vi "Create Case Structure.vi"(6 "Mouse Position":T1, 7 "User VI Ref":refnum<vi>, 8 "Is Multi-select?":bool, 9 "Remaining Items":refnum<vi>[](array[refnum]), 10 "Affected Items":T8, 11 "Menu Refnum":refnum<k9>) -> (3 "Menu Items To Add":T2[](array[typedef]))   [LabVIEW 2024]
doc: "This VI is part of a plug-in for modifying the LabVIEW shortcut menus. This is the builder VI which is called when the shortcut menu is built. It tells LabVIEW which shortcut menu items to add to the menu."
uses:
  <resource>/plugins/PopupMenus/support/Shortcut Menu Item Definition.ctl
  <resource>/plugins/PopupMenus/support/Transaction Control.ctl
  <resource>/plugins/PopupMenus/support/Position In Menu.ctl
  <resource>/plugins/PopupMenus/support/Relative Position.ctl
  <resource>/plugins/PopupMenus/support/Checkmark Status.ctl
  <resource>/plugins/PopupMenus/support/Enabled Menu Item Status.ctl
  <vilib>/Utility/miscctls.llb/LVPositionTypeDef.ctl
panel:
  # "Rules a popup plug-in must follow:\n* This VI's file name must match the file name of the LLB -- only the file extensions should be different.\n* This VI must have debugging disabled or it will be ignored as a plug-in.\n* For all menu items, \"tag suffix + file name of this VI\" must be less than 240 characters.\n* You can disconnect the \"Affected Items\" from the typedef to make the plug-in load faster. The typedef is only there to assist you in keeping this VI and the execution VI using to the same type.\n* All controls on this panel except \"Affected Items\" are locked to prevent accidental edits. Do not change the types or the names of controls other than the elements inside the \"Affected Items\" cluster.\n* See Context Help for more information on the individual controls."
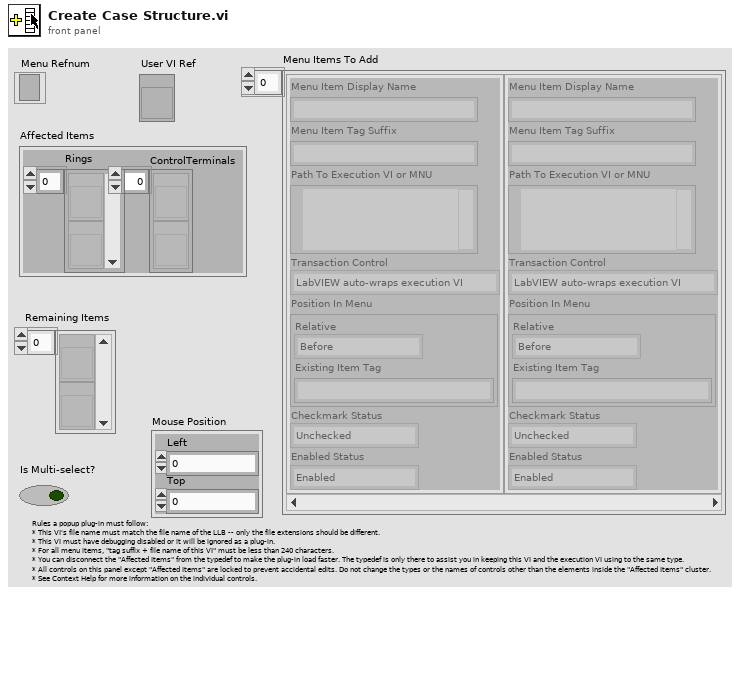
[diagram p1: front panel]
types:
  T1 = typedef "LVPositionTypeDef.ctl" = cluster{"Left":i32, "Top":i32}
  T2 = typedef "Shortcut Menu Item Definition.ctl" = cluster{"Menu Item Display Name":string, "Menu Item Tag Suffix":string, "Path To Execution VI or MNU":path, "Transaction Control":T3, "Position In Menu":T4, "Checkmark Status":T6, "Enabled Status":T7}
  T3 = typedef "Transaction Control.ctl" = enum8{"LabVIEW auto-wraps execution VI", "Execution VI will define if needed"}
  T4 = typedef "Position In Menu.ctl" = cluster{"Relative":T5, "Existing Item Tag":string}
  T5 = typedef "Relative Position.ctl" = enum8{"Before", "Instead of", "After", "Into Submenu"}
  T6 = typedef "Checkmark Status.ctl" = enum8{"Unchecked", "Checked"}
  T7 = typedef "Enabled Menu Item Status.ctl" = enum8{"Enabled", "Disabled"}
  T8 = cluster{"Rings":refnum<vi>[], "ControlTerminals":refnum<vi>[]}
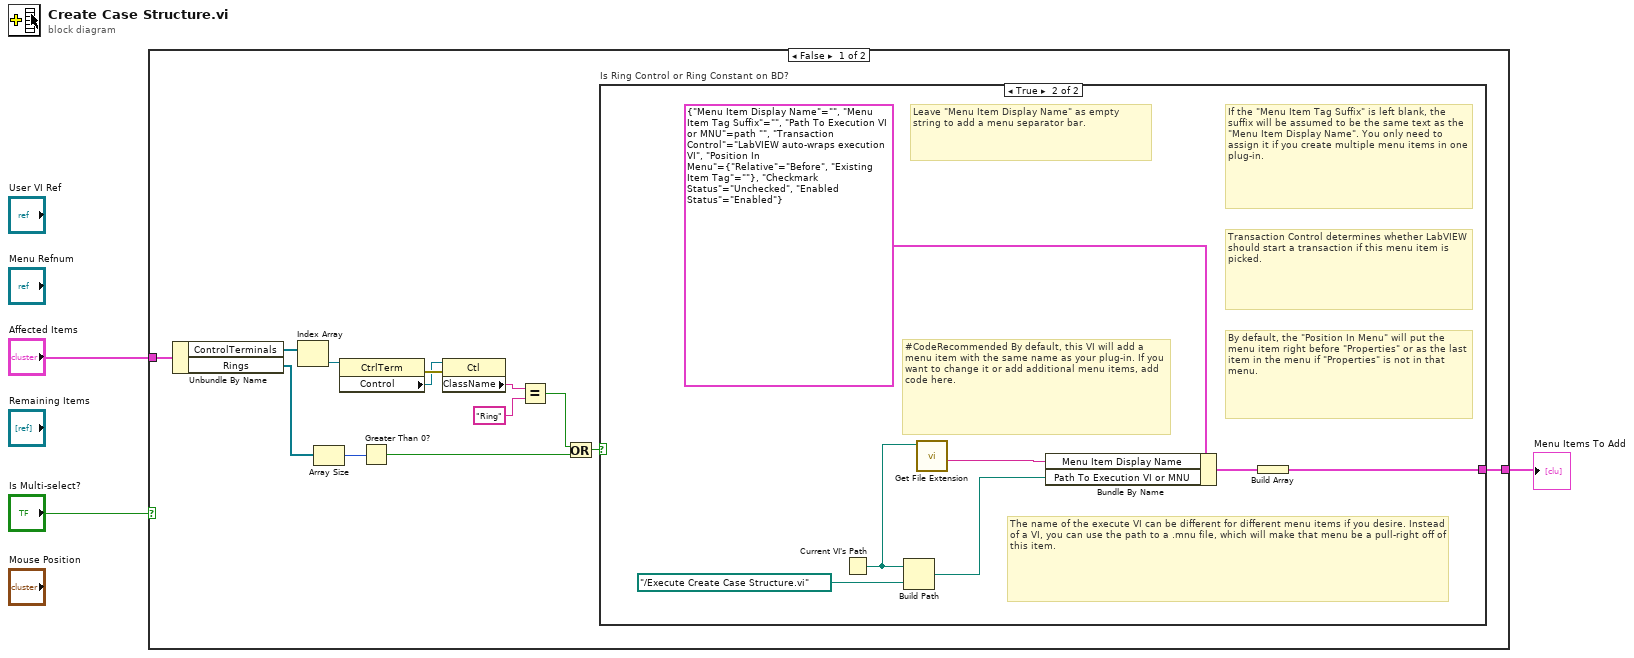
[diagram p0: block diagram]
diagram:
  n1 = case shown="False" "Is Multi-select?" {
    tunnel: "Affected Items" -> [w15 _]
    tunnel: [w16 _] -> w1
    frame False {
      n2 = Unbundle By Name(w15) -> ("ControlTerminals"=w14:refnum<vi>[], "Rings"=w12:refnum<vi>[])
      n3 = Index Array(array=w14) -> (element=w9:refnum<vi>)  [unwired: 1 in]
      n4 = Array Size(array=w12) -> (size(s)=w11:i32)
      n5 = property class="CtrlTerm"(reference=w9) -> (error out=w8:errorcluster, "Control"=w7:refnum<vi>)  [unwired: 1 in, 1 out]
      n6 = Greater Than 0?(x=w11) -> (x > 0?=w10:bool)
      n7 = property class="Ctl"(reference=w7, error in=w8) -> ("ClassName"=w6:string)  [unwired: 2 out]
      n8 = Equal?(x=w6, y="Ring") -> (x = y?=w4:bool)
      n9 = Or(x=w4, y=w10) -> (x .or. y?=w13:bool)
      n10 = case "Is Ring Control or Ring Constant on BD?" shown="True" w13 {
        tunnel: [_ w17] -> w16
        frame False {
        }
        frame True {
          # "Transaction Control determines whether LabVIEW should start a transaction if this menu item is picked."
          # "#CodeRecommended By default, this VI will add a menu item with the same name as your plug-in. If you want to change it or add additional menu items, add code here."
          # "Leave \"Menu Item Display Name\" as empty string to add a menu separator bar."
          # "If the \"Menu Item Tag Suffix\" is left blank, the suffix will be assumed to be the same text as the \"Menu Item Display Name\". You only need to assign it if you create multiple menu items in one plug-in."
          # "By default, the \"Position In Menu\" will put the menu item right before \"Properties\" or as the last item in the menu if \"Properties\" is not in that menu."
          # "The name of the execute VI can be different for different menu items if you desire. Instead of a VI, you can use the path to a .mnu file, which will make that menu be a pull-right off of this item."
          n11 = Current VI's Path() -> (path=w19:path)
          n12 = Build Path(base path=w19, name or relative path=path "../Execute Create Case Structure.vi" ("execute path")) -> (appended path=w22:path)
          n13 = call <vilib>:"Get File Extension.vi"("file"=w19) -> ("filename without extension"=w18:string)  [unwired: 6 in, 4 out]
          n14 = Bundle By Name(cluster=T2 {"Menu Item Display Name"="", "Menu Item Tag Suffix"="", "Path To Execution VI or MNU"=path "", "Transaction Control"=enum."LabVIEW auto-wraps execution VI", "Position In Menu"={"Relative"=enum."Before", "Existing Item Tag"=""}, "Checkmark Status"=enum."Unchecked", "Enabled Status"=enum."Enabled"} ("Cluster"), "Menu Item Display Name"=w18, "Path To Execution VI or MNU"=w22) -> (w20:T2)
          n15 = Build Array(w20) -> (w17:T2[])
        }
      }
    }
    frame True {
    }
  }
  "Menu Items To Add" <- w1
